vi "hello.vi"   [LabVIEW 2022 SP3]
types:
  T1 = enum16{"open", "replace", "create", "open or create", "replace or create", "replace or create with confirmation"}
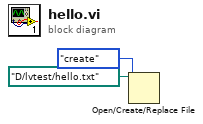
[diagram p0: block diagram]
diagram:
  n1 = Open/Create/Replace File(file path (use dialog)=path "D:/lvtest/hello.txt", operation (0:open)=T1."create") -> ()  [unwired: 4 in, 3 out]
